vi "JSON-ClusterForInstructionsDB.vi"(8 "error in (no error)":errorcluster, 11 "Payload":string) -> (0 "error out":errorcluster, 3 "Cluster Out":T1(array[cluster]))   [LabVIEW 2013]
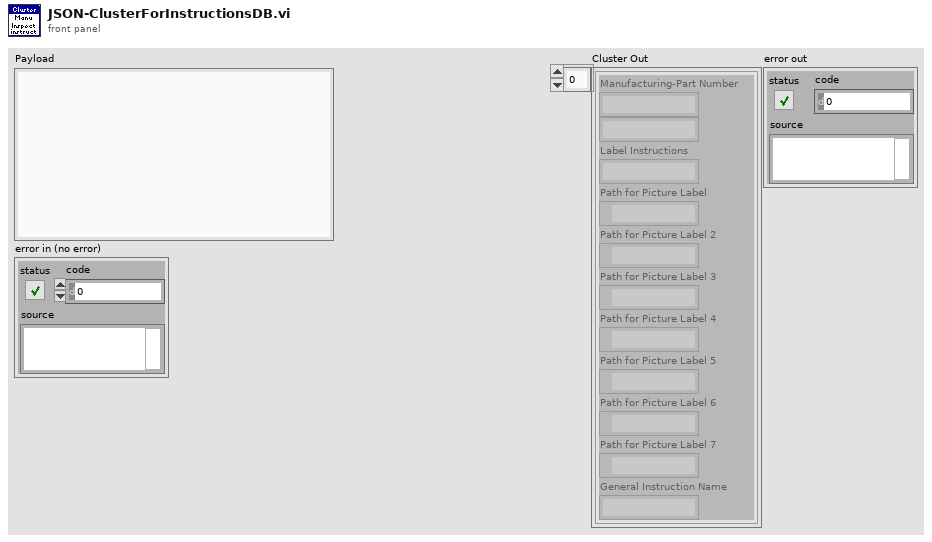
[diagram p1: front panel]
types:
  T1 = cluster{"Manufacturing-Part Number":string, string, "Label Instructions":string, "Path for Picture Label":path, "Path for Picture Label 2":path, "Path for Picture Label 3":path, "Path for Picture Label 4":path, "Path for Picture Label 5":path, "Path for Picture Label 6":path, "Path for Picture Label 7":path, "General Instruction Name":string}[]
  T2 = cluster{"General Process Step 1":string, "General Process Step 2":string, "General Process Step 3":string, "General Process Step 4":string, "General Process Step 5":string, "General Process Step 6":string}
  T3 = cluster{"Manufacturing-Part Number":string, "Array of Cluster Data":cluster{"Label Instructions":string, "Path for Picture Label":path, "Path for Picture Label 2":path, "Path for Picture Label 3":path, "Path for Picture Label 4":path, "Path for Picture Label 5":path, "Path for Picture Label 6":path, "Path for Picture Label 7":path}[], "General Instruction Name":string}
  T4 = cluster{"Label Instructions":string, "Path for Picture Label":path, "Path for Picture Label 2":path, "Path for Picture Label 3":path, "Path for Picture Label 4":path, "Path for Picture Label 5":path, "Path for Picture Label 6":path, "Path for Picture Label 7":path}[]
  T5 = cluster{"Manufacturing-Part Number":string, string, "Label Instructions":string, "Path for Picture Label":path, "Path for Picture Label 2":path, "Path for Picture Label 3":path, "Path for Picture Label 4":path, "Path for Picture Label 5":path, "Path for Picture Label 6":path, "Path for Picture Label 7":path, "General Process Step 1":string}
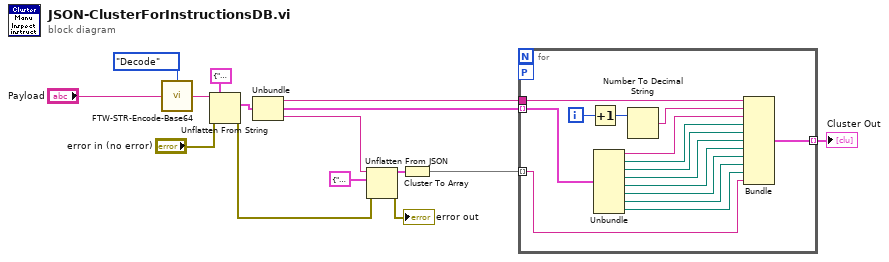
[diagram p0: block diagram]
diagram:
  n1 = call "FTW-STR-Encode-Base64.vi"("Input"="Payload", "Direction"=enum16{"Encode", "Decode"}."Decode") -> ("Output"=w13:string)
  n2 = Unflatten From String(type=T3 {"Manufacturing-Part Number"="", "Array of Cluster Data"=[], "General Instruction Name"=""} ("cluster"), binary string=w13, error in (no error)="error in (no error)") -> (value=w12:T3, error out=w3:errorcluster)  [unwired: 2 in, 1 out]
  n3 = Unbundle(w12) -> ("Manufacturing-Part Number"=w9:string, "Array of Cluster Data"=w10:T4, "General Instruction Name"=w6:string)
  n4 = Unflatten From JSON(JSON string=w6, type and defaults=T2 {"General Process Step 1"="", "General Process Step 2"="", "General Process Step 3"="", "General Process Step 4"="", "General Process Step 5"="", "General Process Step 6"=""}, error in (no error)=w3) -> (value=w2:T2, error out=→"error out":errorcluster)  [unwired: 4 in]
  n5 = Cluster To Array(cluster=w2) -> (array=w1:string[])
  n6 = for {
    tunnel: w10 -> [w30] mode=indexing
    tunnel: w9 -> [w29]
    workers-P: _ -> [_]
    tunnel: [w19] -> w7 mode=indexing
    tunnel: w1 -> [w16] mode=indexing
    i -> [w18]
    n7 = Increment(x=w18) -> (x+1=w17:i32)
    n8 = Unbundle(w30) -> ("Label Instructions"=w27:string, "Path for Picture Label"=w26:path, "Path for Picture Label 2"=w25:path, "Path for Picture Label 3"=w24:path, "Path for Picture Label 4"=w23:path, "Path for Picture Label 5"=w22:path, "Path for Picture Label 6"=w21:path, "Path for Picture Label 7"=w20:path)
    n9 = Number To Decimal String(number=w17) -> (decimal integer string=w28:string)  [unwired: 1 in]
    n10 = Bundle("Manufacturing-Part Number"=w29, w28, "Label Instructions"=w27, "Path for Picture Label"=w26, "Path for Picture Label 2"=w25, "Path for Picture Label 3"=w24, "Path for Picture Label 4"=w23, "Path for Picture Label 5"=w22, "Path for Picture Label 6"=w21, "Path for Picture Label 7"=w20, "General Process Step 1"=w16) -> (w19:T5)  [unwired: 1 in]
  }
  "Cluster Out" <- w7
